vi "MakeScreenshotOnlyGraph.vi"(7 "error in (no error)":errorcluster, 9 "String in":refnum<vi>, 10 "XYGraph Refnum":refnum<vi>) -> (0 "error out":errorcluster)   [LabVIEW 2018]
doc: "This example captures an image of the front panel of a VI and saves the image to a JPG, PNG, or BMP file."
panel:
  out "Image path":path
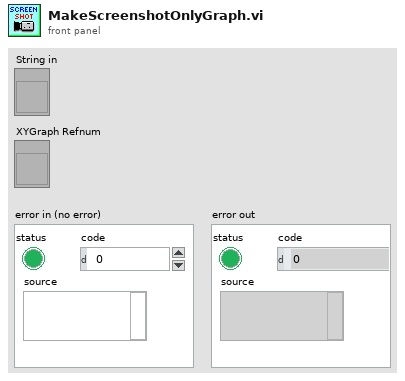
[diagram p1: front panel]
types:
  T1 = typedef "imagedata.ctl" = cluster{"image type":i32, "image depth":i32, "image":u8[], "mask":u8[], "colors":u32[], "Rectangle":cluster{"left":i16, "top":i16, "right":i16, "bottom":i16}}
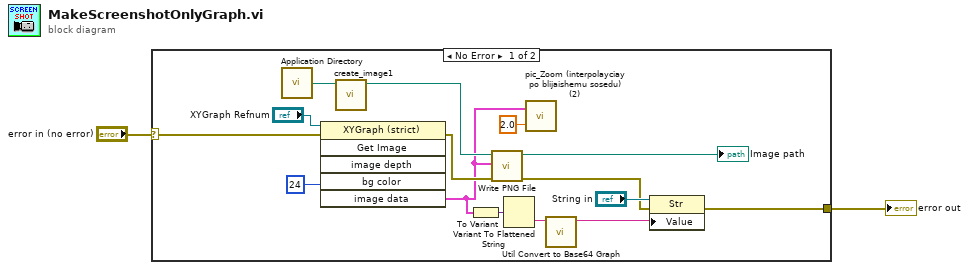
[diagram p0: block diagram]
diagram:
  n1 = case shown="No Error" "error in (no error)" {
    selector: "error in (no error)" -> [w6 w18]
    tunnel: [w9 w18] -> w2
    frame No Error {
      n2 = call <vilib>:"Application Directory.vi"() -> ("Application Directory"=w8:path)
      n3 = invoke class="XYGraph (strict)" method="Get Image"(reference="XYGraph Refnum", error in=w6, "bg color"=24 ("Image Depth")) -> (error out=w17:errorcluster, "image data"=w3:T1)  [unwired: 3 in, 4 out]
      n4 = call "create_image1.vi"("base path"=w8) -> ("path"=w7:path)  [unwired: 9 in, 1 out]
      n5 = To Variant(anything=w3) -> (Variant=w12:variant)
      n6 = call <vilib>:"Write PNG File.vi"("error in (no error)"=w17, "image data"=w3, "path to PNG file"=w7) -> ("error out"=w10:errorcluster, "path"=→"Image path":path)  [unwired: 7 in]
      n7 = Variant To Flattened String(Variant=w12) -> (data string=w13:string)  [unwired: 1 out]
      n8 = call "pic_Zoom (interpolayciay po blijaishemu sosedu) (2).vi"("Zoom"=2.0, "image data IN"=w3) -> ()  [unwired: 1 in, 1 out]
      n9 = call "Util Convert to Base64 Graph.vi"("String"=w13) -> ("Base64 String"=w14:string)  [unwired: 10 in]
      n10 = property on="Property Node" class="Str"(reference="String in", error in=w10, "Value"=w14) -> (error out=w9:errorcluster)  [unwired: 1 out]
    }
    frame Error {
    }
  }
  "error out" <- w2
